vi "SetDigitalFilterControl.vi"(8 "Error In":errorcluster, 9 "Digital Filter Control":T1, 10 "Channel (1 or 2)":u8 min=1 max=2 step=1, 11 "Keithley 6482 In":refnum<visa-resource-name>) -> (0 "Error Out":errorcluster, 3 "Keithley 6482 Out":refnum<visa-resource-name>)   [LabVIEW 2009, in "Keithley-6482-Visa.lvlib"]
uses:
  <instrlib>/Keithley-6482-Visa9.0/Keithley-6482-Visa.lvlib
  <instrlib>/Keithley-6482-Visa9.0/Public/Controls/DigitalFilterControl.ctl
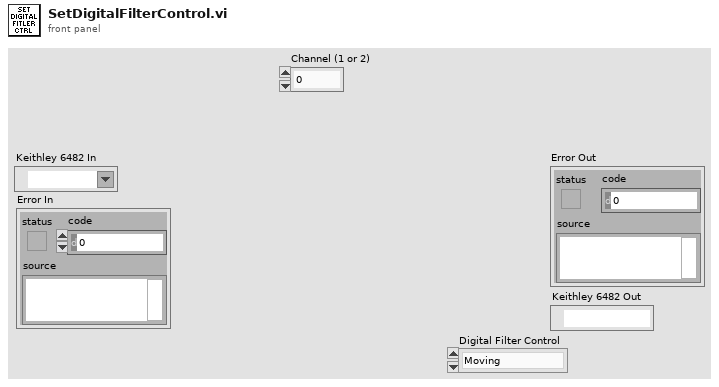
[diagram p1: front panel]
types:
  T1 = typedef "Keithley-6482-Visa.lvlib/DigitalFilterControl.ctl" = enum16{"Moving", "Repeat"}
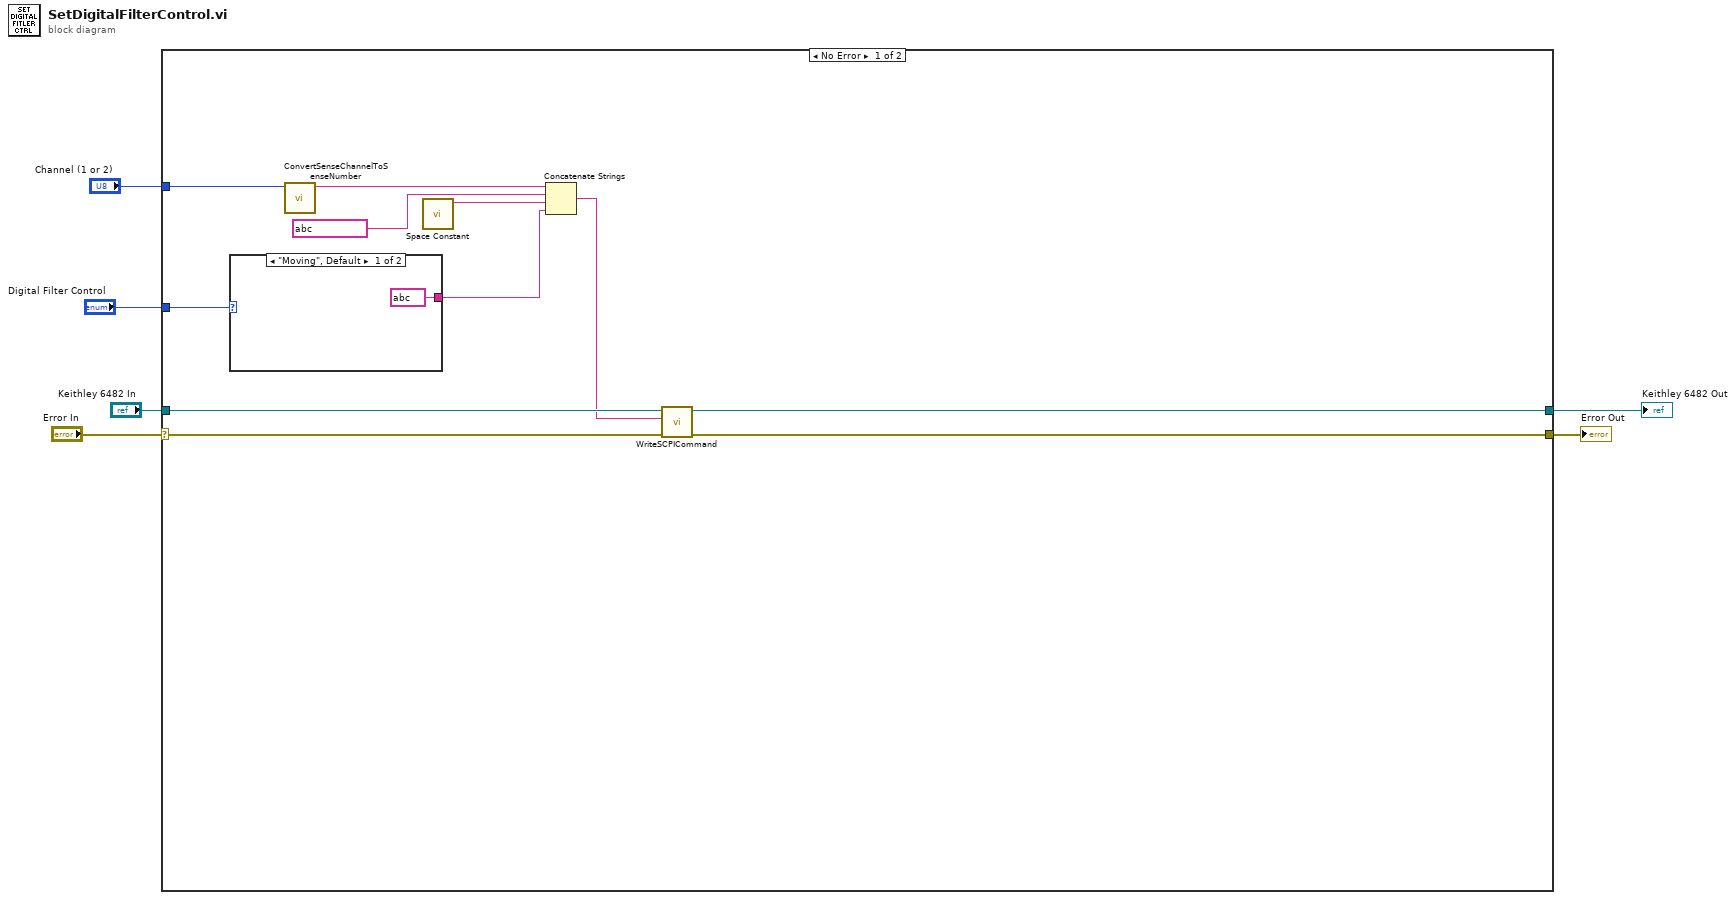
[diagram p0: block diagram]
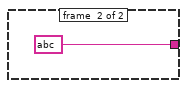
[diagram p2: hidden frame]
diagram:
  n1 = case shown="No Error" "Error In" {
    selector: "Error In" -> [w17 w20]
    tunnel: "Keithley 6482 In" -> [w16 w21]
    tunnel: [w9 w20] -> w4
    tunnel: [w10 w21] -> w3
    tunnel: "Channel (1 or 2)" -> [w15 _]
    tunnel: "Digital Filter Control" -> [w8 _]
    frame #0 {
      n2 = case shown="\"Moving\", Default" w8 {
        tunnel: [string ? string ?] -> w7
        frame #0 {
        }
        frame #1 {
        }
      }
      n3 = call <instrlib>:"ConvertSenseChannelToSenseNumber.vi"("Channel (1 or 2)"=w15) -> ("Sense Number"=w14:string)  [unwired: 10 in]
      n4 = call <vilib>:"Space Constant.vi"() -> ("String"=w12:string)
      n5 = Concatenate Strings(w14, string ? ("string"), w12, w7) -> (w11:string)
      n6 = call <instrlib>:"WriteSCPICommand.vi"("Error In"=w17, "SCPI Command"=w11, "Keithley 6482 In"=w16) -> ("Error Out"=w9:errorcluster, "Keithley 6482 Out"=w10:refnum<visa-resource-name>)  [unwired: 7 in]
    }
    frame #1 {
    }
  }
  "Error Out" <- w4
  "Keithley 6482 Out" <- w3
